vi "修改登录密码.vi"(8 "新密码":string, 9 "旧密码":string, 10 "登录名":string, 11 "数据库连接引用":T1) -> (0 "error out":errorcluster)   [LabVIEW 2013, in "数据库操作.lvclass"]
uses:
  <vilib>/addons/database/Connection.llb/Conn ObjectReference.ctl
  <vilib>/addons/database/Connection.llb/Conn Execute.vi
  <vilib>/addons/database/NI_Database_API.lvlib
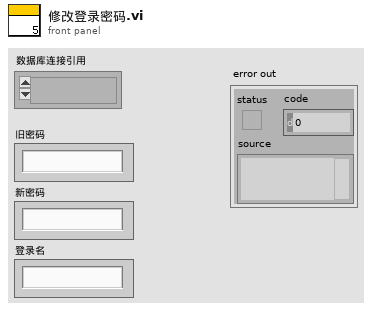
[diagram p1: front panel]
types:
  T1 = typedef "NI_Database_API.lvlib/Conn ObjectReference.ctl" = refnum<k1>
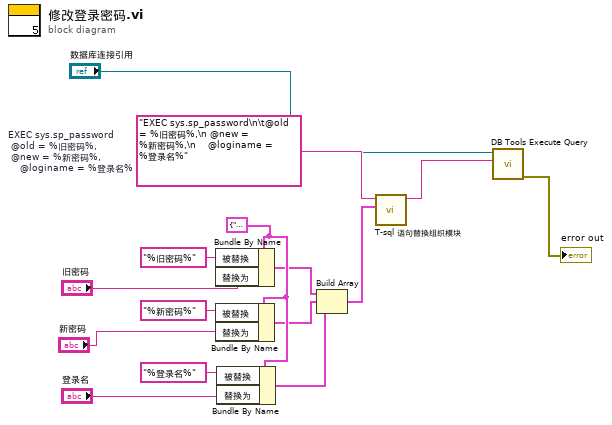
[diagram p0: block diagram]
diagram:
  w14 = cluster{"被替换":string, "替换为":string} {"被替换"="", "替换为"=""} ("替换单元")
  w15 = "EXEC sys.sp_password\n\t@old = %旧密码%,\n @new = %新密码%,\n    @loginame = %登录名%"  # EXEC sys.sp_password 	@old = %旧密码%,  @new = %新密码%,     @loginame = %登录名%
  n1 = Bundle By Name(cluster=w14, "被替换"="%旧密码%", "替换为"="旧密码") -> (w10:cluster{"被替换":string, "替换为":string})
  n2 = Bundle By Name(cluster=w14, "被替换"="%新密码%", "替换为"="新密码") -> (w9:cluster{"被替换":string, "替换为":string})
  n3 = Bundle By Name(cluster=w14, "被替换"="%登录名%", "替换为"="登录名") -> (w8:cluster{"被替换":string, "替换为":string})
  n4 = Build Array(w10, w9, w8) -> (w7:cluster{"被替换":string, "替换为":string}[])
  n5 = call "T-sql 语句替换组织模块.vi"("替换项"=w7, "T-sql 模板"=w15) -> ("T-sql"=w6:string)  [unwired: 8 in, 1 out]
  n6 = call-poly <vilib>:"DB Tools Execute Query.vi"("SQL query"=w6, "connection reference"="数据库连接引用") -> ("error out"=→"error out":errorcluster)  [unwired: 6 in, 1 out]
